vi "Bld_versions.get.vi"(8 "error in":errorcluster, 11 "Build Specs":refnum<vi>[](array[refnum])) -> (0 "error out":errorcluster, 3 "Bld_versions":T2(array[cluster]))   [LabVIEW 2025]
uses:
  <vilib>/AppBuilder/AB_API_Simple/Build Specification Version.ctl
  <vilib>/AppBuilder/AB_API_Simple/NI_App_Builder_API.lvlib
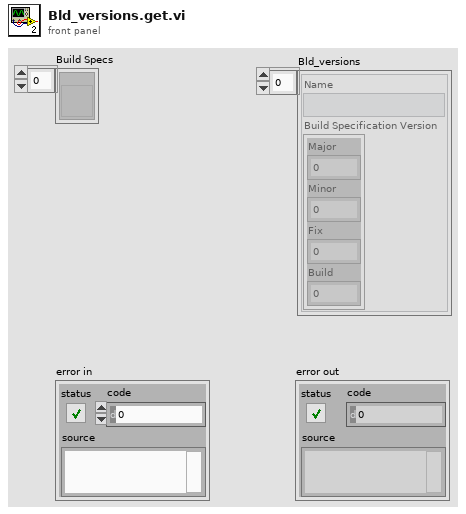
[diagram p1: front panel]
types:
  T1 = typedef "NI_App_Builder_API.lvlib/Build Specification Version.ctl" = cluster{"Major":u16, "Minor":u16, "Fix":u16, "Build":u16}
  T2 = cluster{"Name":string, "Build Specification Version":T1}[]
  T3 = cluster{"Name":string, "Build Specification Version":T1}
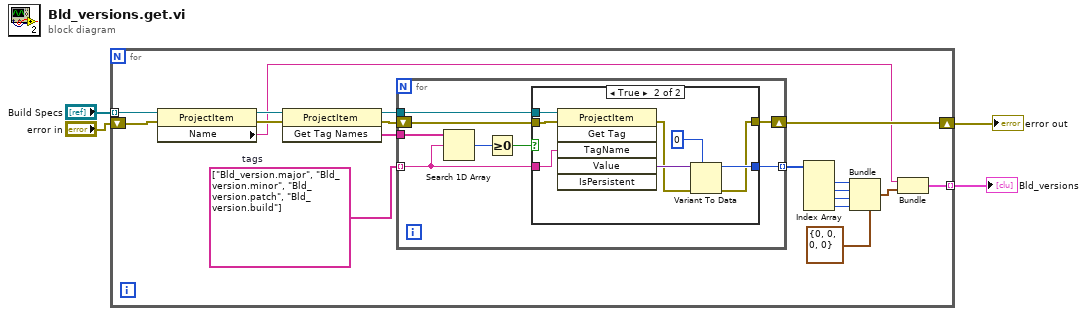
[diagram p0: block diagram]
diagram:
  n1 = for {
    tunnel: "Build Specs" -> [w6] mode=indexing
    shift-right: [w19] -> w1
    shift-left: "error in" -> [w18]
    tunnel: [w7] -> w2 mode=indexing
    w8 = string[] ["Bld_version.major", "Bld_version.minor", "Bld_version.patch", "Bld_version.build"]  # tags
    n2 = property class="ProjectItem"(reference=w6, error in=w18) -> (reference out=w17:refnum<vi>, error out=w16:errorcluster, "Name"=w9:string)
    n3 = invoke class="ProjectItem" method="Get Tag Names"(reference=w17, error in=w16) -> (reference out=w21:refnum<vi>, error out=w20:errorcluster, "Get Tag Names"=w22:string[])  [unwired: 1 in]
    n4 = for {
      tunnel: w22 -> [w30]
      tunnel: w8 -> [w26] mode=indexing
      tunnel: w21 -> [w27]
      shift-right: [w24] -> w19
      shift-left: w20 -> [w25]
      tunnel: [w23] -> w15 mode=indexing
      n5 = Search 1D Array(1D array=w30, element=w26) -> (index of element=w29:i32)  [unwired: 1 in]
      n6 = Greater Or Equal To 0?(x=w29) -> (x >= 0?=w28:bool)
      n7 = case shown="True" w28 {
        tunnel: w27 -> [_ w39]
        tunnel: w26 -> [_ w38]
        tunnel: w25 -> [w31 w37]
        tunnel: [w31 w32] -> w24
        tunnel: [_ w35] -> w23
        frame False {
        }
        frame True {
          n8 = invoke class="ProjectItem" method="Get Tag"(reference=w39, error in=w37, "TagName"=w38) -> (error out=w33:errorcluster, "Value"=w36:variant)  [unwired: 3 in, 4 out]
          n9 = Variant To Data(error in=w33, type=u32 0, Variant=w36) -> (data=w35:u32, error out=w32:errorcluster)
        }
      }
    }
    n10 = Index Array(array=w15) -> (element #1=w13:u32, element #2=w14:u32, element #3=w12:u32, element #4=w11:u32)  [unwired: 4 in]
    n11 = Bundle(cluster=T1 {"Major"=0, "Minor"=0, "Fix"=0, "Build"=0} ("Build Specification Version"), "Major"=w13, "Minor"=w14, "Fix"=w12, "Build"=w11) -> (w10:T1)
    n12 = Bundle("Name"=w9, "Build Specification Version"=w10) -> (w7:T3)  [unwired: 1 in]
  }
  "Bld_versions" <- w2
  "error out" <- w1
